vi "UMB_Arbiter.vi"(11 "Behavior Data":T1=[{"Goodness"=[0, 0, 0, 0, 0, 0, 0, 0, 0, 0, 0, 0, 0, 0, 0], "Velocity"=[0, 0, 0, 0, 0, 0, 0, 0, 0, 0, 0, 0, 0, 0, 0], "Weight"=0}]) -> (1 "prop":i8, 2 "rudder":i32)   [LabVIEW 2012]
uses:
  NINJA Code/Tugboat/Robo_Programs/behaviorData_t.ctl
  NINJA Code/Tugboat/Robo_Programs/behaviorOutput_t.ctl
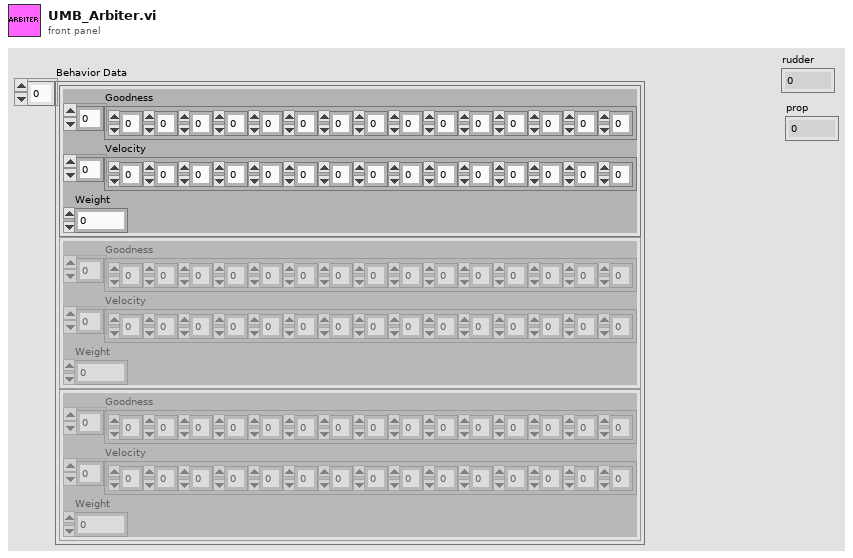
[diagram p1: front panel]
types:
  T1 = typedef "behaviorData_t.ctl" = T2[]
  T2 = typedef "behaviorOutput_t.ctl" = cluster{"Goodness":i8[], "Velocity":i8[], "Weight":i8}
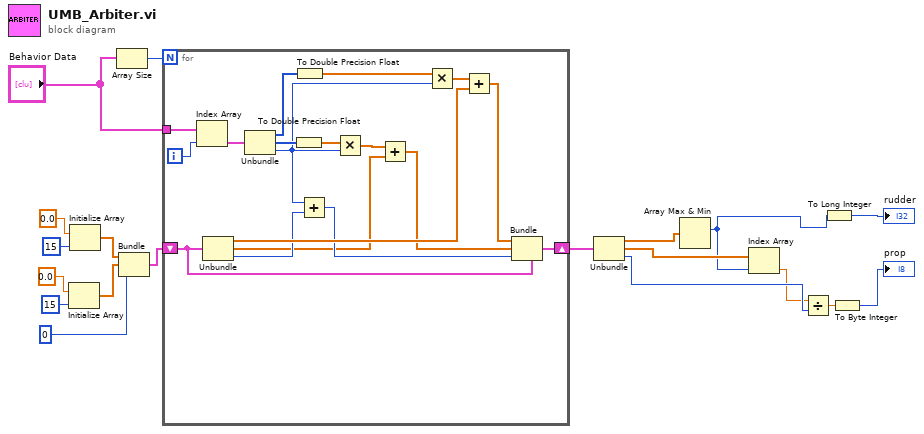
[diagram p0: block diagram]
diagram:
  n1 = Initialize Array(0.0 ("element"), 15 ("dimension size")) -> (w3:dbl[])
  n2 = Initialize Array(0.0 ("element"), 15 ("dimension size")) -> (w4:dbl[])
  n3 = Array Size(array="Behavior Data") -> (size(s)=w19:i32)
  n4 = Bundle(w4, w3, 0) -> (w1:cluster{dbl[], dbl[], i32})  [unwired: 1 in]
  n5 = for {
    N: w19 -> [_]
    shift-right: [w32] -> w17
    shift-left: w1 -> [w33]
    tunnel: "Behavior Data" -> [w36]
    i -> [w37]
    n6 = Index Array(array=w36, index=w37) -> (element=w35:T2)
    n7 = Unbundle(w33) -> (w30:dbl[], w23:dbl[], w28:i32)
    n8 = Unbundle(w35) -> ("Goodness"=w34:i8[], "Velocity"=w26:i8[], "Weight"=w25:i8)
    n9 = To Double Precision Float(number=w26) -> (double precision float=w21:dbl[])
    n10 = To Double Precision Float(number=w34) -> (double precision float=w20:dbl[])
    n11 = Add(x=w25, y=w28) -> (x+y=w27:i32)
    n12 = Multiply(x=w21, y=w25) -> (x*y=w24:dbl[])
    n13 = Add(x=w24, y=w23) -> (x+y=w22:dbl[])
    n14 = Multiply(x=w20, y=w25) -> (x*y=w31:dbl[])
    n15 = Add(x=w31, y=w30) -> (x+y=w29:dbl[])
    n16 = Bundle(cluster=w33, w29, w22, w27) -> (w32:cluster{dbl[], dbl[], i32})
  }
  n17 = Unbundle(w17) -> (w16:dbl[], w15:dbl[], w14:i32)
  n18 = Array Max & Min(array=w16) -> (max index (indices)=w9:i32)  [unwired: 3 out]
  n19 = Index Array(array=w15, index=w9) -> (element=w13:dbl)
  n20 = Divide(x=w13, y=w14) -> (x/y=w12:dbl)
  n21 = To Long Integer(number=w9) -> (32bit integer=→"rudder":i32)
  n22 = To Byte Integer(number=w12) -> (8bit integer=→"prop":i8)
